vi "macro_Debouncer_Execute.vi"   [LabVIEW 2019, in "Trajectory_Library.lvlib"]
uses:
  Trajectory_Library.lvlib
  Enum/DEBOUNCER_TYPE_ENUM.ctl
types:
  T1 = typedef "Trajectory_Library.lvlib/DEBOUNCER_TYPE_ENUM.ctl" = enum16{"Rising", "Falling", "Both"}
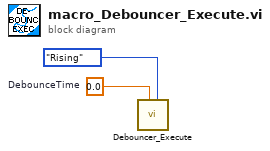
[diagram p0: block diagram]
diagram:
  w2 = 0.0  # DebounceTime
  n1 = call "Debouncer_Execute.vi"("DebounceType"=DEBOUNCER_TYPE_ENUM."Rising", "DebounceTime"=w2) -> ()  [unwired: 8 in, 2 out]
